vi "Constants and GUIDs.vi"() -> ()   [LabVIEW 2013, in "Engine Simulation Toolkit Shared.lvlib"]
doc: "Use this Global VI to access the GUIDs assigned to the page resources of the Custom Device."
uses:
  Engine Simulation Toolkit Shared.lvlib
  Channel.ctl
panel:
  in  "Tab Control":T1(tab)=enum."Constants"
  in  "GUID.Faulting":string="6883F70B-FB69-09B6-41C0-1E5693DBDC1F"
  in  "GUID.Main Disabled":string="C14D209F-F3F6-FCFA-378D-B2711864B4FD"
  in  "GUID.Dir Speed Sensors":string="D53C092C-9273-F5F9-5AE3-78F432D1B155"
  in  "GUID.Dir Speed Sensor":string="5C2C81B2-8355-59B7-A406-02E5DB4E456B"
  in  "GUID.Knock Sensor":string="B616CE42-FE35-D019-E31C-CC10104017BC"
  in  "GUID.Knock Cylinder":string="C77A6EA3-6053-41F6-7CAC-B8F8B0136829"
  in  "GUID.Knock Sensors":string="CDA1C3C4-9193-F2AC-CAE4-3B5D99F75781"
  in  "GUID.Digital Pattern":string="2FB2125B-0883-7010-1B0B-48E566B666E8"
  in  "GUID.Event Capture":string="C87D327C-5609-23E4-5EAA-39DFCD73A8FF"
  in  "GUID.Timing Measurement":string="CDBB0560-26A4-40BA-B1F0-7BA06DDA70DE"
  in  "GUID.Status":string="80DE2635-1DC5-B67A-CA46-E31C1EC1F9C0"
  in  "GUID.Event Measurements":string="0BE9E2FF-E808-70B8-FCAF-CB020D0DBBCB"
  in  "GUID.Generations":string="24C897C1-180F-B7BE-A9FB-811BEBABCC68"
  in  "GUID.APU Commands":string="09792357-1468-7EF4-AB1C-5DDCB9432D68"
  in  "GUID.APU State":string="F1CEE36E-E483-4565-3A3E-AB06893FB67A"
  in  "GUID.Timing":string="E9F52131-D7A3-8DA7-B764-23B3FB65988F"
  in  "GUID.APU":string="4F5791A4-43CD-7687-46C2-FCD7BD4FAF58"
  in  "GUID.Digital Patterns":string="D7284ECD-E3C7-6DB8-B02B-2A9122E191AC"
  in  "GUID.Analog Replays":string="D4A7CD23-71B6-3ACA-56B4-CEA5E66B1FBE"
  in  "GUID.Analog Replay":string="45FB52C5-8FE1-5ED8-79EB-4D665F5CC299"
  in  "GUID.APUs":string="E5C01B3B-7C22-64FD-D709-1CD1836F7D3B"
  in  "GUID.Sect Del Prot":string="120667F2-0B41-D791-AB55-B102D2164F36"
  in  "GUID.Chan Del Prot":string="CAB9E886-793C-6FFE-E190-E227CA9E28A0"
  in  "GUID.Main Enabled":string="7baffd2f-e585-46fb-ac82-fc4feb050845"
  in  "Constant.Faulting":string="Faulting"
  in  "Constant.Pick Tooth Source":string="Select an item..."
  in  "Constant.Dir Speed Sensors":string="Directional Speed"
  in  "Constant.Knock Sensors":string="Knock"
  in  "Constant.Pick FPGA resource":string="Select an item..."
  in  "Constant.invalid bitfile":string="None detected"
  in  "Constant.ConfirmDelete":string="Confirm delete configuration"
  in  "Constant.ChangeBItfile":string="Changing the bitfile path will delete all configuration information. Proceed?"
  in  "Constant.RemoveBitfile":string="Removing the bitfile path will delete all configuration information. Proceed?"
  in  "Constant.Status":string="Status"
  in  "Constant.Waveforms":string="Waveforms"
  in  "Constant.Thresholding":string="Thresholding"
  in  "Constant.Event Timing":string="Event Timing"
  in  "Constant.Measurements":string="Measurements"
  in  "Constant.Digital Patterns":string="Digital Patterns"
  in  "Constant.Analog Replays":string="Analog Replays"
  in  "Constant.Generations":string="Generations"
  in  "Constant.State":string="State"
  in  "Constant.Commands":string="Commands"
  in  "Constant.not present":string="- not added -"
  in  "ChanList.DirSpeedSensor":T2[](array[typedef])=[{"Name"="Td", "Units"="uS", "Default"=5.0, "Description"="Delay time before a pulse is generated after passing a tooth center."}, {"Name"="Tf", "Units"="uS", "Default"=45.0, "Description"="Duration of pulse generation during forward rotation."}, {"Name"="Tr", "Units"="uS", "Default"=90.0, "Description"="Duration of pulse generation during reverse rotation."}]
  in  "ChanList.KnockSensor":T2[](array[typedef])=[{"Name"="Amplitude", "Units"="V", "Default"=1.0, "Description"="Amplitude of the always present low frequency signal from the knock sensor."}]
  in  "ChanList.KnockCylinder":T2[](array[typedef])=[{"Name"="Probability", "Units"="%", "Default"=0.0, "Description"="Set a value between zero and one hundred for the probability of a knock occuring."}, {"Name"="Amplitude", "Units"="V", "Default"=5.0, "Description"="Amplitude of the knock signal, should it occur."}, {"Name"="Trigger Angle", "Units"="deg", "Default"=0.0, "Description"="Angle the knock occurs if triggered."}]
  in  "ChanList.EventCapture":T2[](array[typedef])=[{"Name"="Start angle", "Units"="deg", "Default"=0.0, "Description"="Cycle angle which the event went from inactive to active. If there was no start angle captured within the measurement window or for a full cycle, the default start angle value is returned instead."}, {"Name"="End angle", "Units"="deg", "Default"=0.0, "Description"="Cycle angle which the event went from active to inactive. If there was no end angle captured within the measurement window or for a full cycle, the default end angle value is returned instead."}, {"Name"="Duration", "Units"="ms", "Default"=0.0, "Description"="Duration of event active time within the measurement window."}]
  in  "ChanList.MeasurementStatus":T2[](array[typedef])=[{"Name"="Stuck active", "Units"="", "Default"=0.0, "Description"="True if the event being measured was active for longer than the configured stuck active limit"}, {"Name"="All active window", "Units"="", "Default"=0.0, "Description"="True if the event being measured was active for an entire measurement window"}, {"Name"="Orphan start edge", "Units"="", "Default"=0.0, "Description"="True if there was an inactive to active edge inside the last measurement window without a corresponding active to inactive edge."}, {"Name"="Orphan end edge", "Units"="", "Default"=0.0, "Description"="True if there was an active to inactive edge inside the last measurement window without a corresponding inactive to active edge."}]
  in  "ChanList.DataReplayVoltage":T2[](array[typedef])=[{"Name"="Enable voltage override", "Units"="", "Default"=0.0, "Description"="A value other than zero enables overriding the analog data replay's preconfigured voltage scaling slope and intercept with the corresponding channel values."}, {"Name"="Voltage slope", "Units"="", "Default"=0.0, "Description"="Slope of the engine speed scaling applied to the analog data replay voltage. Voltage value = (slope * FPGA_Engine_Speed + offset) * replay data. \nImportant notes: Replay data is always normalized to full scale range of the analog output DAC. FPGA_Engine_Speed is equal to RPM * (1/60) * (1/40M) * 2^16."}, {"Name"="Voltage intercept", "Units"="", "Default"=0.0, "Description"="Offset of the engine speed scaling applied to the analog data replay voltage. Voltage value = (slope * FPGA_Engine_Speed + offset) * replay data. \nImportant notes: Replay data is always normalized to full scale range of the analog output DAC. FPGA_Engine_Speed is equal to RPM * (1/60) * (1/40M) * 2^16."}]
  in  "ChanList.Offset":T2[](array[typedef])=[{"Name"="Offset", "Units"="deg", "Default"=0.0, "Description"="This value is added to the engine's rotational position."}]
  in  "ChanList.Status Chans":T2[](array[typedef])=[{"Name"="Status code", "Units"="", "Default"=0.0, "Description"="Status code of the custom device. A negative value indicates failure. A positive value indicates warning."}, {"Name"="Loop duration", "Units"="ns", "Default"=0.0, "Description"="Duration of the custom device loop in nanoseconds. This can be monitored to measure performance relative to the desired loop rate."}, {"Name"="Late count", "Units"="", "Default"=0.0, "Description"="Number of times the custom device loop has gone late."}]
  in  "ChanList.APU Commands":T2[](array[typedef])=[{"Name"="Desired Speed", "Units"="RPM", "Default"=0.0, "Description"="Engine speed requested from the angle processing unit. This value may be coerced slightly, and acceleration may be applied to this value. Observe the actual speed status channel to see the actual speed the angle processing unit is using."}, {"Name"="Position Reset", "Units"="", "Default"=0.0, "Description"="A value other than zero commands the angle processing unit to reset to its initial position.\nWARNING: This snaps the angle processing unit position and will cause undefined behavior of output generations for a short time. For example, snapping position could cause a large instantaneous position change resulting in knock simulation generating the knock for several cylinders simultaneously. It is only recommended to reset position when the ECU under test is rebooting.\n"}]
  in  "ChanList.APU State":T2[](array[typedef])=[{"Name"="Crank Angle", "Units"="deg", "Default"=0.0, "Description"="The angle processing unit's simulated position in terms of crank degrees."}, {"Name"="Cycle Angle", "Units"="deg", "Default"=0.0, "Description"="The angle processing unit's simulated position in terms of cycle degrees."}, {"Name"="Actual Speed", "Units"="RPM", "Default"=0.0, "Description"="The actual speed value the angle processing unit is using to calculate positions. Note that the resultant positions will slowly accumulate error as compared to the rotational speed due to numerical representation."}]
  in  "ChanList.DigPtrnFaultingOut":T2[](array[typedef])=[{"Name"="Valid settings", "Units"="", "Default"=0.0, "Description"="Indicates the fault settings are valid and will be applied upon trigger."}]
  in  "ChanList.DigPtrnFaultingIn":T2[](array[typedef])=[{"Name"="Command", "Units"="", "Default"=0.0, "Description"="0: On rising edge of trigger, set the digital pattern to finish faulting after its next or current fault insertion is finished. \n1: On rising edge of trigger, remove the specified tooth # from the pattern for the specified number of rotations.  \n2: On rising edge of trigger, force the digital output low between start angle and stop angle for the specified number of rotations. \n3: On rising edge of trigger, force the digital output high between start angle and stop angle for the specified number of rotations."}, {"Name"="Trigger", "Units"="", "Default"=0.0, "Description"="Ignored if valid settings is false."}, {"Name"="Rotations", "Units"="", "Default"=0.0, "Description"="Up to 16. 0 means indefinitely until faulting is commanded to finish."}, {"Name"="Start angle", "Units"="deg", "Default"=0.0, "Description"="Rotational position to begin faulting."}, {"Name"="Stop angle", "Units"="deg", "Default"=0.0, "Description"="Rotational position to end faulting."}, {"Name"="Tooth to remove", "Units"="", "Default"=0.0, "Description"="Tooth number of the pattern to remove during faulting. Teeth are 1 indexed from the begining of the rotation (crank or cycle) to the end."}]
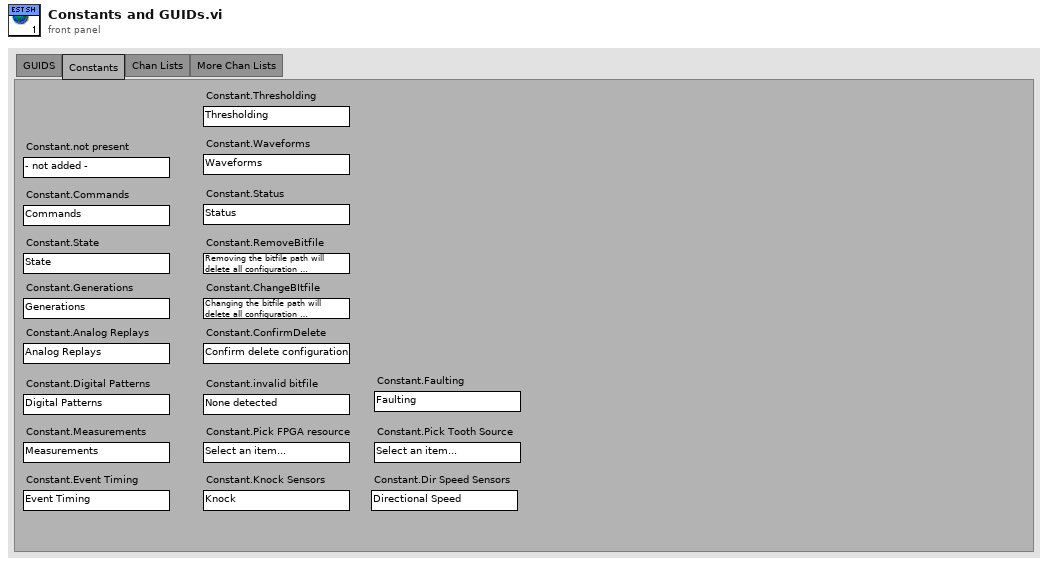
[diagram p1: front panel]
types:
  T1 = enum32{"GUIDS", "Constants", "Chan Lists", "More Chan Lists"}
  T2 = typedef "Engine Simulation Toolkit Shared.lvlib/Channel.ctl" = cluster{"Name":string, "Units":string, "Default":dbl, "Description":string}
diagram:
